vi "create file name.vi"(8 "error in (no error)":errorcluster, 11 "Log File in":refnum<class "Log File.lvclass">) -> (0 "error out":errorcluster, 3 "Log File out":refnum<class "Log File.lvclass">)   [LabVIEW 2018, in "Log File.lvclass"]
uses:
  Log File.lvclass
  Log File.lvclass/Log File.ctl
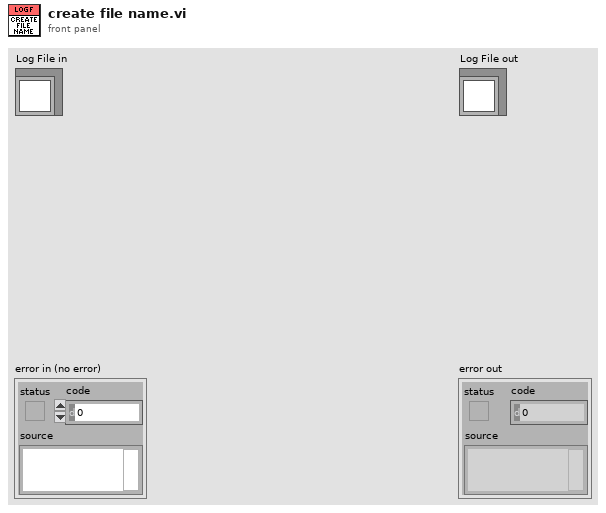
[diagram p1: front panel]
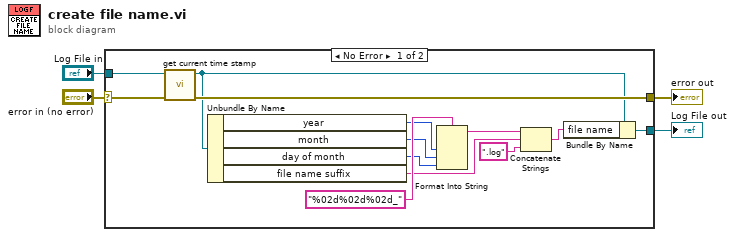
[diagram p0: block diagram]
diagram:
  n1 = case shown="No Error" "error in (no error)" {
    selector: "error in (no error)" -> [w11 w18]
    tunnel: [w10 w18] -> w3
    tunnel: [w17 w19] -> w1
    tunnel: "Log File in" -> [w12 w19]
    frame No Error {
      n2 = call "get current time stamp.vi"("error in (no error)"=w11, "Log File in"=w12) -> ("error out"=w10:errorcluster, "Log File out"=w9:refnum<class "Log File.lvclass">)  [unwired: 8 in]
      n3 = Unbundle By Name(w9) -> ("year"=w8:i32, "month"=w7:i32, "day of month"=w6:i32, "file name suffix"=w5:string)
      n4 = Format Into String(format string="%02d%02d%02d_", w8, w7, w6) -> (resulting string=w15:string)  [unwired: 2 in, 1 out]
      n5 = Concatenate Strings(w15, w5, ".log" ("string")) -> (w13:string)
      n6 = Bundle By Name(cluster=w9, "file name"=w13) -> (w17:refnum<class "Log File.lvclass">)
    }
    frame Error {
    }
  }
  "error out" <- w3
  "Log File out" <- w1
